vi "5-2 clusters.vi"() -> ()   [LabVIEW 2015]
panel:
  out "Numeric":dbl
  out "Boolean 2":bool
  in  "stop":bool
  out "Small Cluster":cluster{"Boolean 1":bool, "Slide Value":dbl}
  out "Modified Cluster":T1 {"Slide" scale=0.0..10.0}
  in  "Cluster":T1 {"Slide" scale=0.0..10.0}
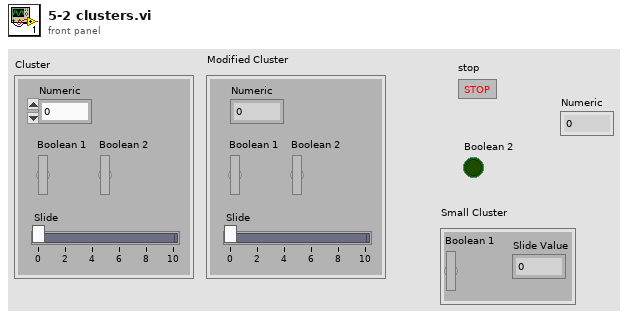
[diagram p1: front panel]
types:
  T1 = cluster{"Numeric":dbl, "Boolean 1":bool, "Boolean 2":bool, "Slide":dbl}
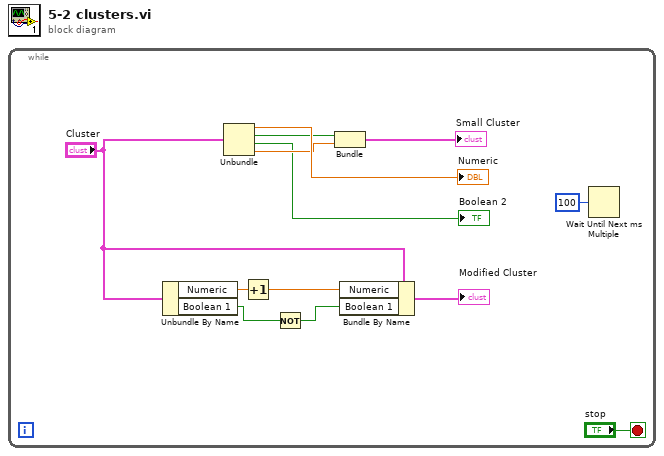
[diagram p0: block diagram]
diagram:
  n1 = while {
    stop <- "stop" stop-if-true
    n2 = Unbundle By Name("Cluster") -> ("Numeric"=w6:dbl, "Boolean 1"=w3:bool)
    n3 = Unbundle("Cluster") -> ("Numeric"=→"Numeric":dbl, "Boolean 1"=w10:bool, "Boolean 2"=→"Boolean 2":bool, "Slide"=w9:dbl)
    n4 = Increment(x=w6) -> (x+1=w5:dbl)
    n5 = Not(x=w3) -> (.not. x?=w4:bool)
    n6 = Bundle("Boolean 1"=w10, "Slide"=w9) -> (→"Small Cluster":cluster{"Boolean 1":bool, "Slide":dbl})  [unwired: 1 in]
    n7 = Bundle By Name(cluster="Cluster", "Numeric"=w5, "Boolean 1"=w4) -> (→"Modified Cluster":T1)
    n8 = Wait Until Next ms Multiple(millisecond multiple=u32 100) -> ()  [unwired: 1 out]
  }
